vi "Acquisition Message Loop.vi"(8 "error in (no error)":errorcluster, 10 "Data Notifier":refnum<notifier>, 11 "Message Queues":T1) -> (0 "error out":errorcluster)   [LabVIEW 2017, in "Acquisition.lvlib"]
doc: "Message loop for handling messages pertaining to the acquisition of data from the hardware."
uses:
  Acquisition.lvlib
  support/Message Queue/All Message Queues.ctl
  support/Message Queue/Message Cluster.ctl
  Hardware Configuration.ctl
  Acquisition State.ctl
  support/Message Queue/Enqueue Message (Single).vi
  <vilib>/Utility/error.llb/Error Cluster From Error Code.vi
  <vilib>/ErrorRing/Error Ring.xnode
  support/Message Queue/Message Queue.lvlib
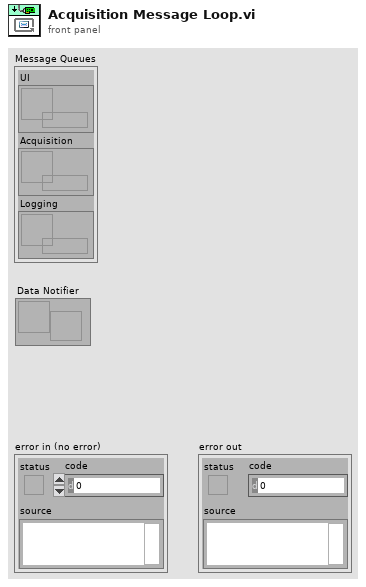
[diagram p1: front panel]
types:
  T1 = typedef "Message Queue.lvlib/All Message Queues.ctl" = cluster{"UI":refnum<queue>, "Acquisition":refnum<queue>, "Logging":refnum<queue>}
  T2 = typedef "Acquisition.lvlib/Hardware Configuration.ctl" = cluster{"Sensor Channels":tag, "Max Input":dbl, "Min Input":dbl, "Sample Rate":dbl, "DAQmx Task":refnum<k21>, "Reference Channels":tag}
  T3 = typedef "Acquisition.lvlib/Acquisition State.ctl" = enum16{"Idle", "Acquiring"}
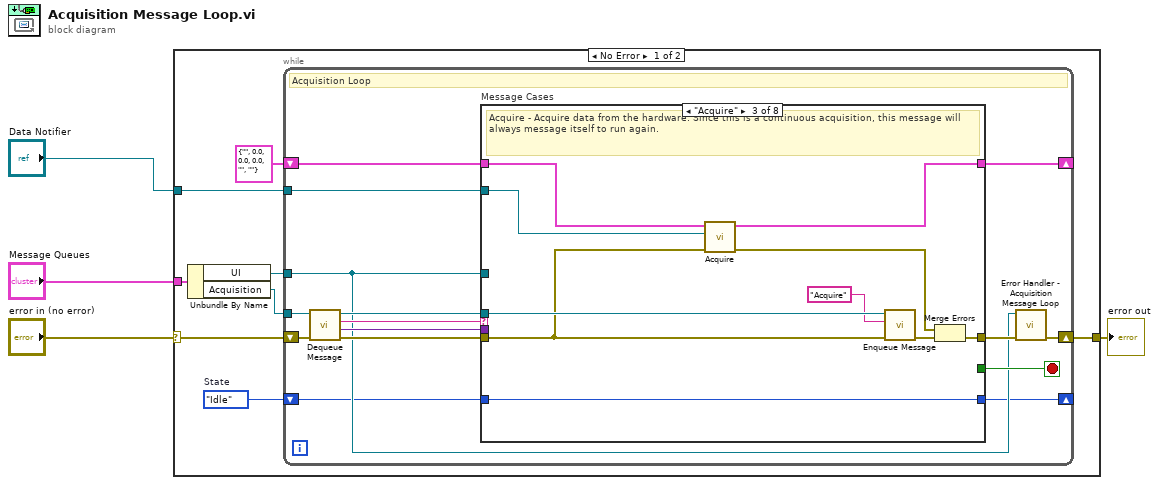
[diagram p0: block diagram]
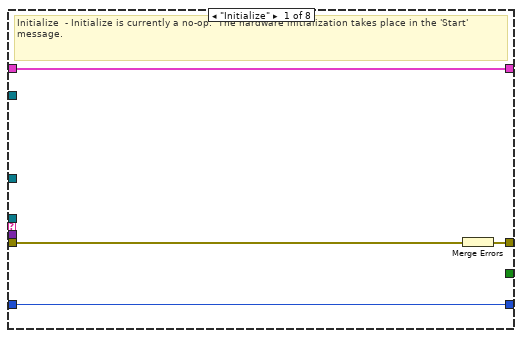
[diagram p2: hidden frame]
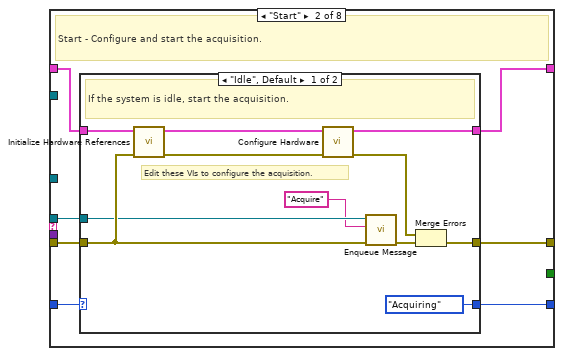
[diagram p3: hidden frame]
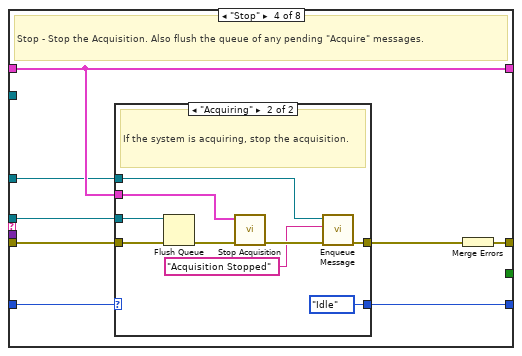
[diagram p5: hidden frame]
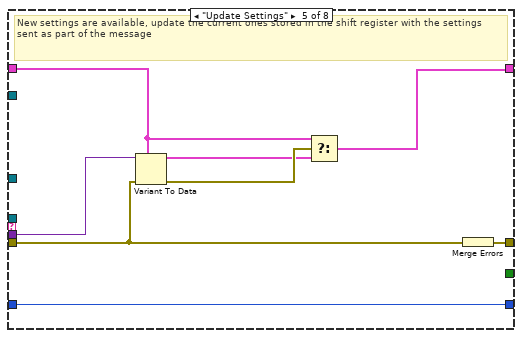
[diagram p7: hidden frame]
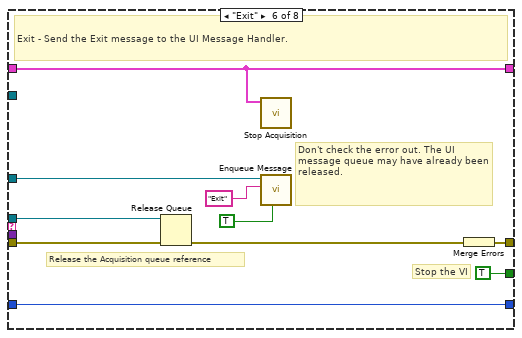
[diagram p8: hidden frame]
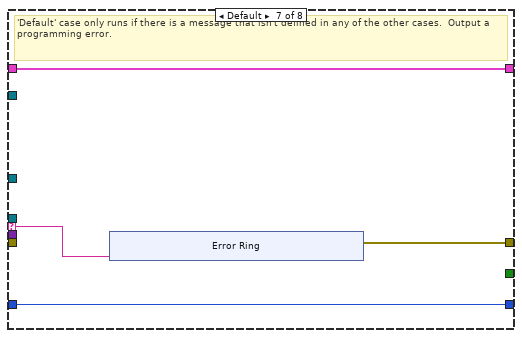
[diagram p9: hidden frame]
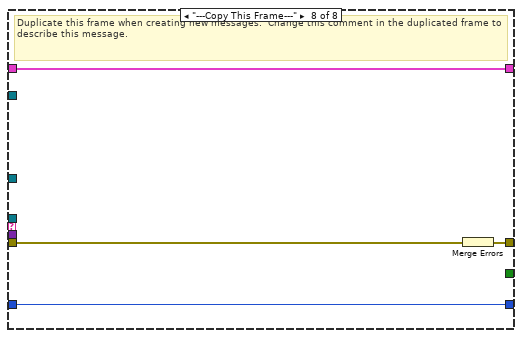
[diagram p10: hidden frame]
diagram:
  n1 = case shown="No Error" "error in (no error)" {
    selector: "error in (no error)" -> [w8 w115]
    tunnel: "Message Queues" -> [w12 _]
    tunnel: [w10 w115] -> w3
    tunnel: "Data Notifier" -> [w6 _]
    frame No Error {
      w5 = Acquisition_State."Idle"  # State
      n2 = Unbundle By Name(w12) -> ("UI"=w7:refnum<queue>, "Acquisition"=w11:refnum<queue>)
      n3 = while {
        tunnel: w11 -> [w19]
        shift-right: [w26] -> _
        shift-left: T2 {"Sensor Channels"="", "Max Input"=0.0, "Min Input"=0.0, "Sample Rate"=0.0, "DAQmx Task"="", "Reference Channels"=""} ("Data Cluster") -> [w27]
        shift-right: [w16] -> w10
        shift-left: w8 -> [w24]
        tunnel: w7 -> [w15]
        tunnel: w6 -> [w18]
        shift-right: [w13] -> _
        shift-left: w5 -> [w14]
        stop <- w25 stop-if-true
        # "Acquisition Loop"
        n4 = call "Dequeue Message.vi"("error in (no error)"=w24, "Message Queue"=w19) -> ("error out"=w23:errorcluster, "Message Data"=w21:variant, "Message"=w22:string, "dup Message Queue"=w20:refnum<queue>)  [unwired: 6 in]
        n5 = case "Message Cases" shown="\"Acquire\"" w22 {
          selector: w22 -> [_ _ _ _ _ _ w102 _]
          tunnel: w20 -> [_ w35 w60 w67 _ w92 _ _]
          tunnel: w23 -> [w30 w36 w59 w69 w83 w96 _ w114]
          tunnel: [w31 w38 w62 w70 w89 w98 w101 w112] -> w17
          tunnel: w27 -> [w29 w37 w56 w68 w85 w91 w103 w113]
          tunnel: [w29 w34 w57 w68 w84 w91 w103 w113] -> w26
          tunnel: [_ _ _ _ _ TRUE _ _] -> w25
          tunnel: w21 -> [_ _ _ _ w88 _ _ _]
          tunnel: w15 -> [_ _ _ w66 _ w97 _ _]
          tunnel: w18 -> [_ _ w54 _ _ _ _ _]
          tunnel: w14 -> [w28 w33 w53 w65 w82 w90 w100 w111]
          tunnel: [w28 w32 w53 w64 w82 w90 w100 w111] -> w13
          frame "Initialize" {
            # "Initialize  - Initialize is currently a no-op.  The hardware initialization takes place in the 'Start' message."
            n6 = Merge Errors(w30) -> (w31:errorcluster)
          }
          frame "Start" {
            # "Start - Configure and start the acquisition."
            n7 = case shown="\"Idle\", Default" w33 {
              selector: w33 -> [_ w50]
              tunnel: [w49 w52] -> w38
              tunnel: w37 -> [w48 w51]
              tunnel: w36 -> [w47 w52]
              tunnel: w35 -> [w45 _]
              tunnel: [w41 w51] -> w34
              tunnel: [Acquisition_State."Acquiring" ("State") w50] -> w32
              frame "Idle", Default {
                # "Edit these VIs to configure the acquisition."
                # "If the system is idle, start the acquisition."
                n8 = call "Initialize Hardware References.vi"("error in (no error)"=w47, "Hardware Resources in"=w48) -> ("error out"=w44:errorcluster, "Hardware Resources out"=w42:T2)  [unwired: 8 in]
                n9 = call "Configure Hardware.vi"("error in (no error)"=w44, "Hardware Resources in"=w42) -> ("error out"=w43:errorcluster, "Hardware Resources out"=w41:T2)  [unwired: 8 in]
                n10 = call-poly "Enqueue Message.vi"("error in (no error)"=w47, "Message"="Acquire", "Message Queue"=w45) -> ("error out"=w46:errorcluster)  [unwired: 7 in, 1 out]
                n11 = Merge Errors(w43, w46) -> (w49:errorcluster)
              }
              frame "Acquiring" {
                # "The system is already acquiring. Ignore the \"Start\" message."
              }
            }
          }
          frame "Acquire" {
            # "Acquire - Acquire data from the hardware. Since this is a continuous acquisition, this message will always message itself to run again."
            n12 = call "Acquire.vi"("error in (no error)"=w59, "Data Notifier"=w54, "Hardware Resources in"=w56) -> ("error out"=w58:errorcluster, "Hardware Resources out"=w57:T2)  [unwired: 7 in]
            n13 = call-poly "Enqueue Message.vi"("error in (no error)"=w59, "Message"="Acquire", "Message Queue"=w60) -> ("error out"=w61:errorcluster)  [unwired: 7 in, 1 out]
            n14 = Merge Errors(w58, w61) -> (w62:errorcluster)
          }
          frame "Stop" {
            # "Stop - Stop the Acquisition. Also flush the queue of any pending \"Acquire\" messages."
            n15 = case shown="\"Acquiring\"" w65 {
              selector: w65 -> [w72 _]
              tunnel: w69 -> [w71 w81]
              tunnel: w68 -> [_ w80]
              tunnel: w67 -> [_ w78]
              tunnel: w66 -> [_ w77]
              tunnel: [w72 Acquisition_State."Idle" ("State")] -> w64
              tunnel: [w71 w75] -> w63
              frame "Idle", Default {
                # "The system is already idle. Ignore the \"Stop\" message."
              }
              frame "Acquiring" {
                # "If the system is acquiring, stop the acquisition."
                n16 = Flush Queue(queue=w78, error in (no error)=w81) -> (error out=w79:errorcluster)  [unwired: 2 out]
                n17 = call "Stop Acquisition.vi"("error in (no error)"=w79, "Hardware Resources in"=w80) -> ("error out"=w76:errorcluster)  [unwired: 9 in]
                n18 = call-poly "Enqueue Message.vi"("error in (no error)"=w76, "Message"="Acquisition Stopped", "Message Queue"=w77) -> ("error out"=w75:errorcluster)  [unwired: 7 in, 1 out]
              }
            }
            n19 = Merge Errors(w63) -> (w70:errorcluster)
          }
          frame "Update Settings" {
            # "New settings are available, update the current ones stored in the shift register with the settings sent as part of the message"
            n20 = Variant To Data(error in=w83, type=w85, Variant=w88) -> (data=w86:T2, error out=w87:errorcluster)
            n21 = Select(t=w85, s=w87, f=w86) -> (s? t:f=w84:T2)
            n22 = Merge Errors(w83) -> (w89:errorcluster)
          }
          frame "Exit" {
            # "Don't check the error out. The UI message queue may have already been released."
            # "Release the Acquisition queue reference"
            # "Stop the VI"
            # "Exit - Send the Exit message to the UI Message Handler."
            n23 = Release Queue(queue=w92, error in (no error)=w96) -> (error out=w93:errorcluster)  [unwired: 1 in, 2 out]
            n24 = call "Stop Acquisition.vi"("Hardware Resources in"=w91) -> ()  [unwired: 10 in, 1 out]
            n25 = call-poly "Enqueue Message.vi"("Priority Message? (F)"=TRUE, "Message"="Exit", "Message Queue"=w97) -> ()  [unwired: 7 in, 2 out]
            n26 = Merge Errors(w93) -> (w98:errorcluster)
          }
          frame Default {
            # "'Default' case only runs if there is a message that isn't defined in any of the other cases.  Output a programming error."
            n27 = xnode "Error Ring"("parameter 0"=w102) -> ("error out"=w101:errorcluster)
          }
          frame "---Copy This Frame---" {
            # "Duplicate this frame when creating new messages.  Change this comment in the duplicated frame to describe this message."
            n28 = Merge Errors(w114) -> (w112:errorcluster)
          }
        }
        n29 = call "Error Handler - Acquisition Message Loop.vi"("error in (no error)"=w17, "Message Queue"=w15) -> ("dup error in"=w16:errorcluster)  [unwired: 8 in, 1 out]
      }
    }
    frame Error {
    }
  }
  "error out" <- w3
